vi "Sysdef.SimpleImport.vi"(7 "Overwrite Existing?":bool=TRUE, 8 "error in (no error)":errorcluster, 10 "SysDef":T1 {"Tree"."Properties"."Type" items=["K_STRING", "K_BOOL", "K_I32", "K_U32", "K_DOUBLE", "K_U64", "K_VARIANT", "K_DEPENDENTFILE", "K_DEPENDENTNODE", "K_DATASOURCENODE", "K_U16", "K_DBLARR", "K_U32ARR", "K_I32ARR", "K_STRINGARR", "K_DICTIONARY", "K_DICTIONARYARR"]}, 11 "NodeID":u64) -> (0 "error out":errorcluster, 3 "NodeID out":u64)   [LabVIEW 2015, in "System Definition Utilities.lvlib"]
uses:
  System Definition Utilities.lvlib
  _Types/SysDef.Export.ctl
  _Types/TreeItem.ctl
  _Types/TreeItem.Info.ctl
  <vilib>/NI Veristand/Custom Device API/Custom Device Channel.ctl
  <vilib>/NI Veristand/Custom Device API/Custom Device Channel Type.ctl
  <vilib>/NI Veristand/Custom Device API/Custom Device Waveform.ctl
  <vilib>/NI Veristand/Custom Device API/Custom Device Waveform DataType.ctl
  _Types/TreeItem.Property.ctl
  NationalInstruments.VeriStand.SystemDefinitionAPI
  NationalInstruments.VeriStand.SystemStorage
  <vilib>/NI Veristand/Custom Device API/Custom Device API.lvlib
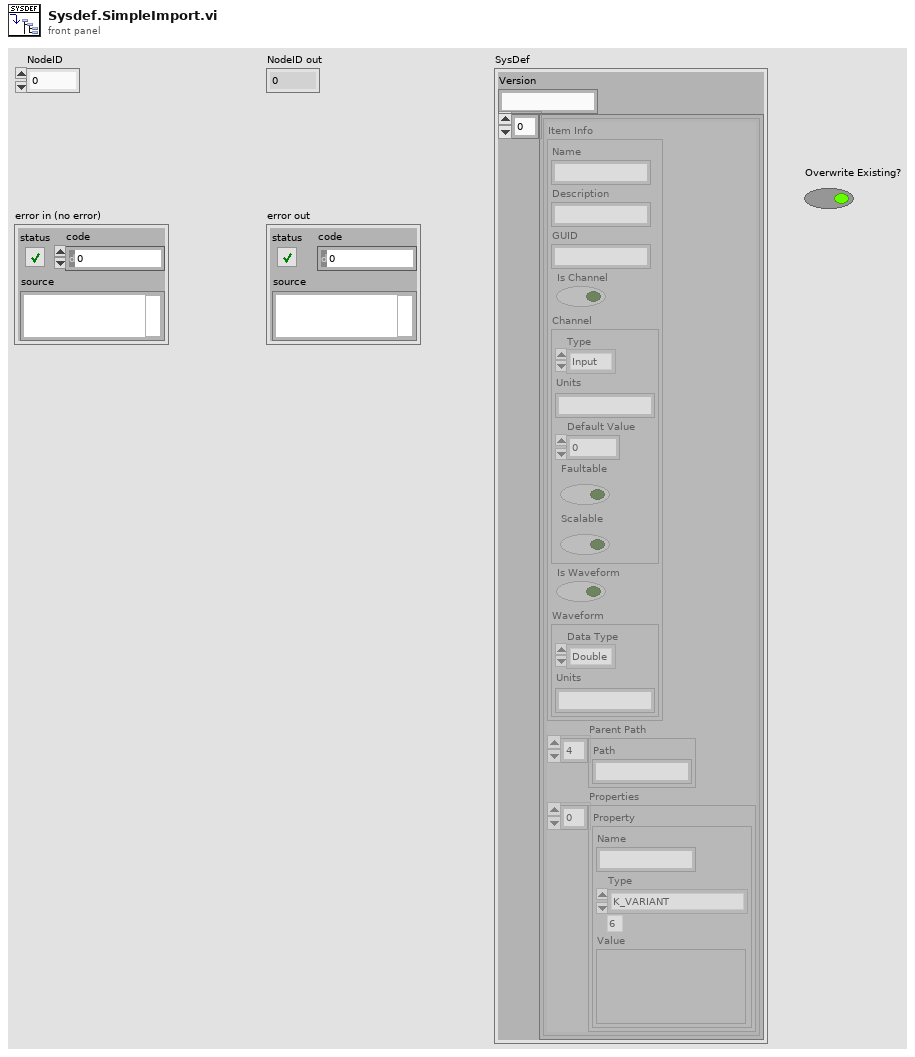
[diagram p1: front panel]
types:
  T1 = typedef "System Definition Utilities.lvlib/SysDef.Export.ctl" = cluster{"Version":string, "Tree":T2[]}
  T2 = typedef "System Definition Utilities.lvlib/TreeItem.ctl" = cluster{"Item Info":T3, "Parent Path":string[], "Properties":T8[]}
  T3 = typedef "System Definition Utilities.lvlib/TreeItem.Info.ctl" = cluster{"Name":string, "Description":string, "GUID":string, "Is Channel":bool, "Channel":T4, "Is Waveform":bool, "Waveform":T6}
  T4 = typedef "Custom Device API.lvlib/Custom Device Channel.ctl" = cluster{"Type":T5, "Units":string, "Default Value":dbl, "Faultable":bool, "Scalable":bool}
  T5 = typedef "Custom Device API.lvlib/Custom Device Channel Type.ctl" = enum16{"Input", "Output"}
  T6 = typedef "Custom Device API.lvlib/Custom Device Waveform.ctl" = cluster{"Data Type":T7, "Units":string}
  T7 = typedef "Custom Device API.lvlib/Custom Device Waveform DataType.ctl" = enum16{"Double", "Complex Double"}
  T8 = typedef "System Definition Utilities.lvlib/TreeItem.Property.ctl" = cluster{"Name":string, "Type":i32, "Value":variant}
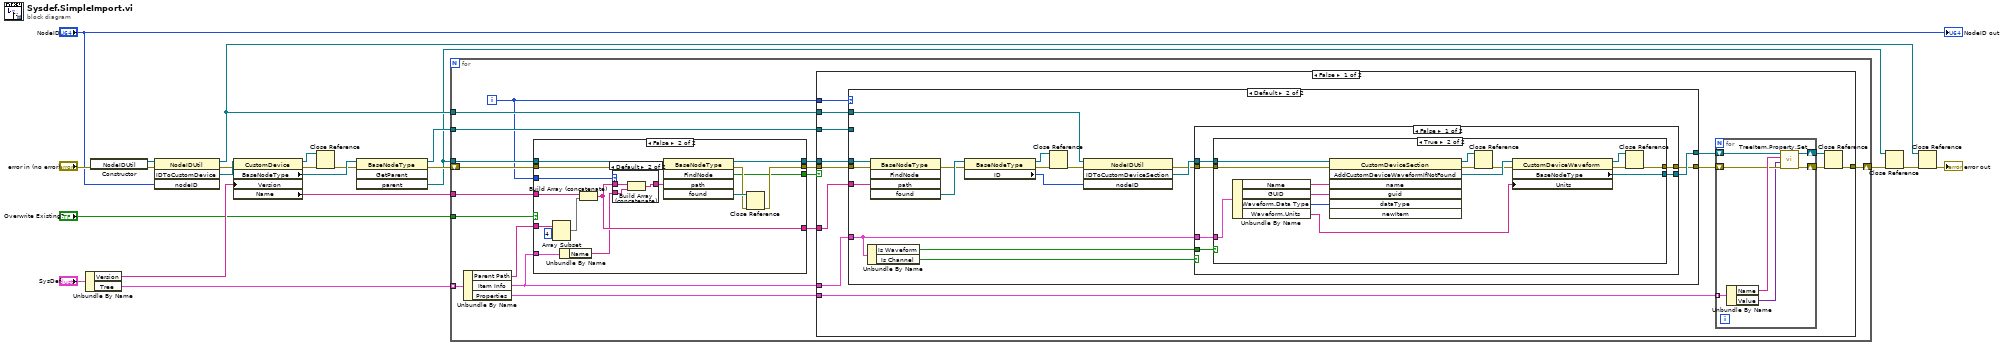
[diagram p0: block diagram]
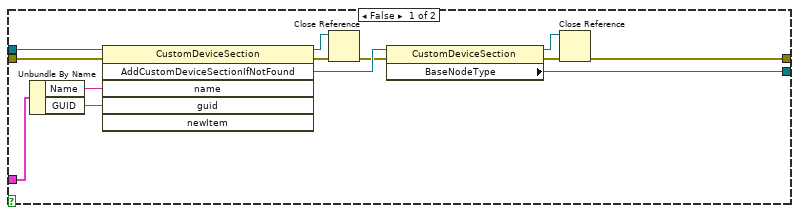
[diagram p3: hidden frame]
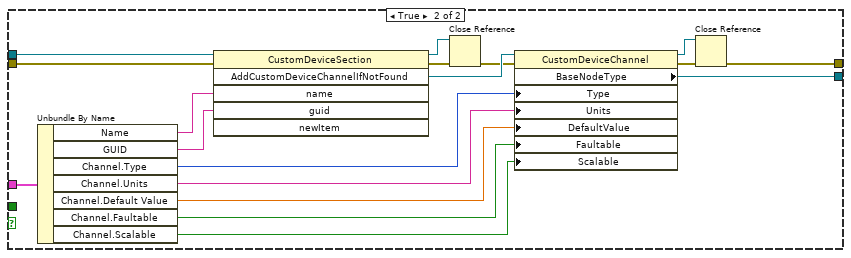
[diagram p4: hidden frame]
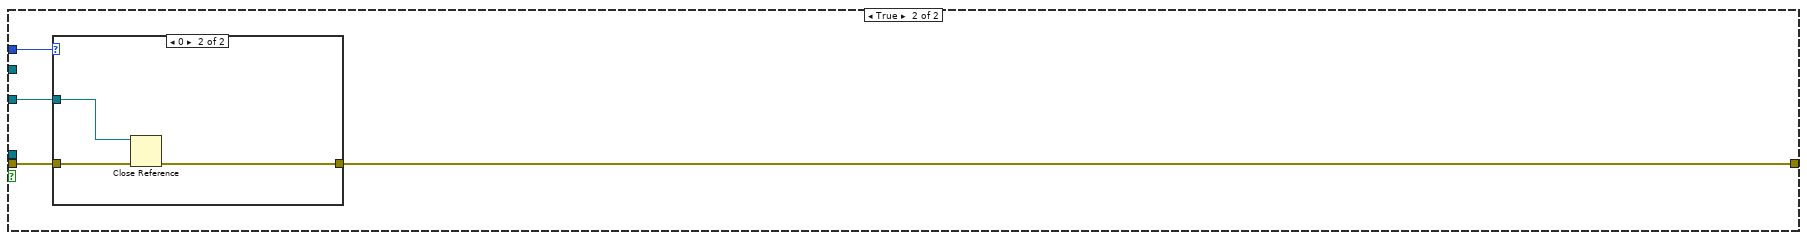
[diagram p5: hidden frame]
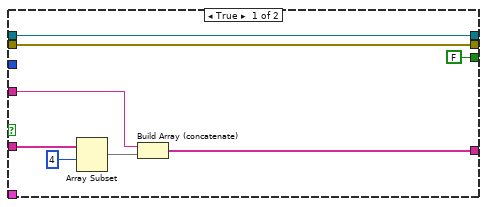
[diagram p7: hidden frame]
diagram:
  n1 = Unbundle By Name("SysDef") -> ("Version"=w19:string, "Tree"=w21:T2[])
  n2 = constructor class="NodeIDUtil"(error in="error in (no error)") -> (reference out=w16:refnum<k24>, error out=w15:errorcluster)  [unwired: 2 in, 1 out]
  n3 = invoke class="NodeIDUtil" method="IDToCustomDevice"(reference=w16, error in=w15, "nodeID"="NodeID") -> (reference out=w2:refnum<k24>, error out=w14:errorcluster, "IDToCustomDevice"=w17:refnum<k24>)  [unwired: 1 in, 1 out]
  n4 = property class="CustomDevice"(reference=w17, error in=w14, "Version"=w19) -> (reference out=w13:refnum<k24>, error out=w11:errorcluster, "BaseNodeType"=w12:refnum<k24>, "Name"=w7:string)
  n5 = Close Reference(reference=w13, error in (no error)=w11) -> (error out=w10:errorcluster)
  n6 = invoke class="BaseNodeType" method="GetParent"(reference=w12, error in=w10) -> (reference out=w8:refnum<k24>, error out=w9:errorcluster, "parent"=w1:refnum<k24>)  [unwired: 2 in, 1 out]
  n7 = for {
    tunnel: w21 -> [w38] mode=indexing
    shift-right: [w35] -> w4
    shift-left: w9 -> [w29]
    tunnel: w8 -> [w34]
    tunnel: w7 -> [w33]
    tunnel: "Overwrite Existing?" -> [w30]
    tunnel: w2 -> [w25]
    tunnel: w1 -> [w24]
    i -> [w23]
    n8 = Unbundle By Name(w38) -> ("Parent Path"=w36:string[], "Item Info"=w31:T3, "Properties"=w37:T8[])
    n9 = case shown="False" w30 {
      tunnel: w36 -> [w144 w160]
      tunnel: w33 -> [w142 w158]
      tunnel: [w141 w156] -> w32
      tunnel: w31 -> [_ w157]
      tunnel: w29 -> [w139 w154]
      tunnel: w24 -> [w140 w152]
      tunnel: [w140 w151] -> w28
      tunnel: [w139 w148] -> w27
      tunnel: [FALSE ("FindNode") w147] -> w26
      tunnel: w23 -> [_ w146]
      frame True {
        n10 = Array Subset(array=w144, index=4) -> (w143:string[])  [unwired: 1 in]
        n11 = Build Array (concatenate)(w142, w143) -> (w141:string[])
      }
      frame False {
        n12 = Array Subset(array=w160, index=4) -> (w159:string[])  [unwired: 1 in]
        n13 = Unbundle By Name(w157) -> ("Name"=w155:string)
        n14 = Build Array (concatenate)(w158, w159) -> (w156:string[])
        n15 = case shown="Default" w146 {
          tunnel: w156 -> [w162 w165]
          tunnel: w155 -> [_ w164]
          tunnel: [w162 w163] -> w153
          frame 0 {
          }
          frame Default {
            n16 = Build Array (concatenate)(w165, w164) -> (w163:string[])
          }
        }
        n17 = invoke class="BaseNodeType" method="FindNode"(reference=w152, error in=w154, "path"=w153) -> (reference out=w151:refnum<k24>, error out=w149:errorcluster, "FindNode"=w147:bool, "found"=w150:refnum<k24>)  [unwired: 2 in, 1 out]
        n18 = Close Reference(reference=w150, error in (no error)=w149) -> (error out=w148:errorcluster)
      }
    }
    n19 = case shown="False" w26 {
      tunnel: w37 -> [w50 _]
      tunnel: w25 -> [w48 _]
      tunnel: [w45 w131] -> w35
      tunnel: w23 -> [w44 w133]
      tunnel: w34 -> [w43 w130]
      tunnel: w32 -> [w42 _]
      tunnel: w31 -> [w41 _]
      tunnel: w28 -> [w40 _]
      tunnel: w27 -> [w39 w132]
      frame False {
        n20 = case shown="Default" w44 {
          tunnel: w39 -> [w53 w67]
          tunnel: [w53 w57] -> w51
          tunnel: [w52 w58] -> w49
          tunnel: w40 -> [_ w70]
          tunnel: w42 -> [_ w69]
          tunnel: w41 -> [_ w59]
          tunnel: w48 -> [_ w63]
          tunnel: w43 -> [w52 _]
          frame 0 {
          }
          frame Default {
            n21 = Unbundle By Name(w59) -> ("Is Waveform"=w56:bool, "Is Channel"=w60:bool)
            n22 = invoke class="BaseNodeType" method="FindNode"(reference=w70, error in=w67, "path"=w69) -> (error out=w65:errorcluster, "found"=w68:refnum<k24>)  [unwired: 2 in, 3 out]
            n23 = property class="BaseNodeType"(reference=w68, error in=w65) -> (reference out=w54:refnum<k24>, error out=w64:errorcluster, "ID"=w66:u64)
            n24 = Close Reference(reference=w54, error in (no error)=w64) -> (error out=w55:errorcluster)
            n25 = invoke class="NodeIDUtil" method="IDToCustomDeviceSection"(reference=w63, error in=w55, "nodeID"=w66) -> (error out=w61:errorcluster, "IDToCustomDeviceSection"=w62:refnum<k24>)  [unwired: 1 in, 2 out]
            n26 = case shown="False" w60 {
              tunnel: w62 -> [w75 w114]
              tunnel: w61 -> [w74 w105]
              tunnel: w59 -> [w71 w113]
              tunnel: [w73 w109] -> w58
              tunnel: [w72 w106] -> w57
              tunnel: w56 -> [w76 _]
              frame False {
                n27 = case shown="True" w76 {
                  tunnel: w75 -> [w86 w100]
                  tunnel: w74 -> [w87 w99]
                  tunnel: [w81 w90] -> w73
                  tunnel: [w77 w92] -> w72
                  tunnel: w71 -> [w85 w98]
                  frame False {
                    n28 = Unbundle By Name(w85) -> ("Name"=w84:string, "GUID"=w83:string)
                    n29 = invoke class="CustomDeviceSection" method="AddCustomDeviceSectionIfNotFound"(reference=w86, error in=w87, "name"=w84, "guid"=w83) -> (reference out=w88:refnum<k24>, error out=w89:errorcluster, "AddCustomDeviceSectionIfNotFound"=w82:refnum<k24>)  [unwired: 2 in, 3 out]
                    n30 = Close Reference(reference=w88, error in (no error)=w89) -> (error out=w80:errorcluster)
                    n31 = property class="CustomDeviceSection"(reference=w82, error in=w80) -> (reference out=w79:refnum<k24>, error out=w78:errorcluster, "BaseNodeType"=w81:refnum<k24>)
                    n32 = Close Reference(reference=w79, error in (no error)=w78) -> (error out=w77:errorcluster)
                  }
                  frame True {
                    n33 = Unbundle By Name(w98) -> ("Name"=w97:string, "GUID"=w96:string, "Waveform.Data Type"=w95:T7, "Waveform.Units"=w91:string)
                    n34 = invoke class="CustomDeviceSection" method="AddCustomDeviceWaveformIfNotFound"(reference=w100, error in=w99, "name"=w97, "guid"=w96, "dataType"=w95) -> (reference out=w103:refnum<k24>, error out=w104:errorcluster, "AddCustomDeviceWaveformIfNotFound"=w102:refnum<k24>)  [unwired: 2 in, 4 out]
                    n35 = Close Reference(reference=w103, error in (no error)=w104) -> (error out=w101:errorcluster)
                    n36 = property class="CustomDeviceWaveform"(reference=w102, error in=w101, "Units"=w91) -> (reference out=w94:refnum<k24>, error out=w93:errorcluster, "BaseNodeType"=w90:refnum<k24>)
                    n37 = Close Reference(reference=w94, error in (no error)=w93) -> (error out=w92:errorcluster)
                  }
                }
              }
              frame True {
                n38 = Unbundle By Name(w113) -> ("Name"=w112:string, "GUID"=w111:string, "Channel.Type"=w110:T5, "Channel.Units"=w118:string, "Channel.Default Value"=w117:dbl, "Channel.Faultable"=w116:bool, "Channel.Scalable"=w115:bool)
                n39 = invoke class="CustomDeviceSection" method="AddCustomDeviceChannelIfNotFound"(reference=w114, error in=w105, "name"=w112, "guid"=w111) -> (reference out=w121:refnum<k24>, error out=w122:errorcluster, "AddCustomDeviceChannelIfNotFound"=w120:refnum<k24>)  [unwired: 2 in, 3 out]
                n40 = Close Reference(reference=w121, error in (no error)=w122) -> (error out=w119:errorcluster)
                n41 = property class="CustomDeviceChannel"(reference=w120, error in=w119, "Type"=w110, "Units"=w118, "DefaultValue"=w117, "Faultable"=w116, "Scalable"=w115) -> (reference out=w108:refnum<k24>, error out=w107:errorcluster, "BaseNodeType"=w109:refnum<k24>)
                n42 = Close Reference(reference=w108, error in (no error)=w107) -> (error out=w106:errorcluster)
              }
            }
          }
        }
        n43 = for {
          shift-right: [w129] -> w46
          shift-left: w51 -> [w124]
          tunnel: w50 -> [w127] mode=indexing
          shift-right: [w126] -> w47
          shift-left: w49 -> [w128]
          n44 = Unbundle By Name(w127) -> ("Name"=w125:string, "Value"=w123:variant)
          n45 = call "TreeItem.Property.Set.vi"("error in (no error)"=w124, "Value"=w123, "Property Name"=w125, "BaseNodeType"=w128) -> ("error out"=w129:errorcluster, "BaseNodeType"=w126:refnum<k24>)  [unwired: 5 in, 1 out]
        }
        n46 = Close Reference(reference=w47, error in (no error)=w46) -> (error out=w45:errorcluster)
      }
      frame True {
        n47 = case shown="0" w133 {
          tunnel: w132 -> [w134 w137]
          tunnel: [w134 w136] -> w131
          tunnel: w130 -> [_ w135]
          frame Default {
          }
          frame 0 {
            n48 = Close Reference(reference=w135, error in (no error)=w137) -> (error out=w136:errorcluster)
          }
        }
      }
    }
  }
  n49 = Close Reference(reference=w1, error in (no error)=w4) -> (error out=w3:errorcluster)
  n50 = Close Reference(reference=w2, error in (no error)=w3) -> (error out=→"error out":errorcluster)
  "NodeID out" <- "NodeID"
